vi "Read Valid Pixels Size.vi"(8 "error in (no error)":errorcluster, 11 "ImageRectifier in":refnum<class "ImageRectifier.lvclass">) -> (0 "error out":errorcluster, 2 "Image Size":T1, 3 "ImageRectifier out":refnum<class "ImageRectifier.lvclass">)   [LabVIEW 2020, in "g_ar_toolkit.image.lvlib" / "ImageRectifier.lvclass"]
uses:
  ImageRectifier.lvclass
  g_ar_toolkit.common/Image Size (Integer).ctl
  ImageRectifier.lvclass/ImageRectifier.ctl
  g_ar_toolkit.common/g_ar_toolkit.common.lvlib
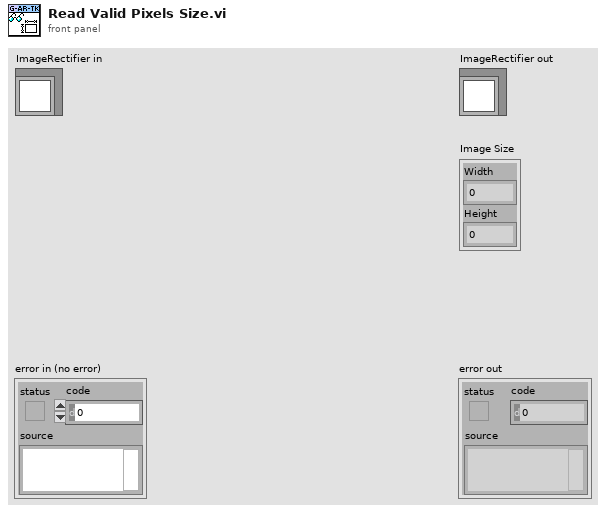
[diagram p1: front panel]
types:
  T1 = typedef "g_ar_toolkit.common.lvlib/Image Size (Integer).ctl" = cluster{"Width":u16, "Height":u16}
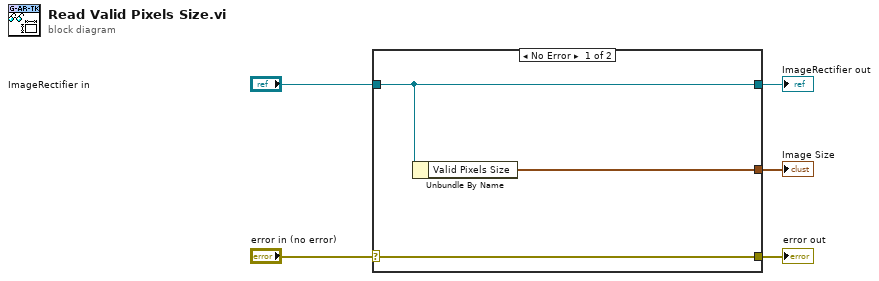
[diagram p0: block diagram]
diagram:
  n1 = case shown="No Error" "error in (no error)" {
    selector: "error in (no error)" -> [w8 w9]
    tunnel: [w8 w9] -> w4
    tunnel: [w7 w10] -> w2
    tunnel: "ImageRectifier in" -> [w7 w10]
    tunnel: [w6 _] -> w1
    frame No Error {
      n2 = Unbundle By Name(w7) -> ("Valid Pixels Size"=w6:T1)
    }
    frame Error {
    }
  }
  "error out" <- w4
  "ImageRectifier out" <- w2
  "Image Size" <- w1
